vi "SelectPage2.vi"(8 "error in (no error)":errorcluster, 11 "Controller in":refnum<class "Controller.lvclass">) -> (0 "error out":errorcluster, 3 "Controller out":refnum<class "Controller.lvclass">)   [LabVIEW 2020, in "Container.lvlib" / "Controller.lvclass"]
uses:
  Controller.lvclass
  Controller.lvclass/Controller.ctl
  Page2/View/View.lvclass
  C:/Users/N Tan/Documents/2-Prototypes/MVC-Multi-Page/iView/iView.lvclass
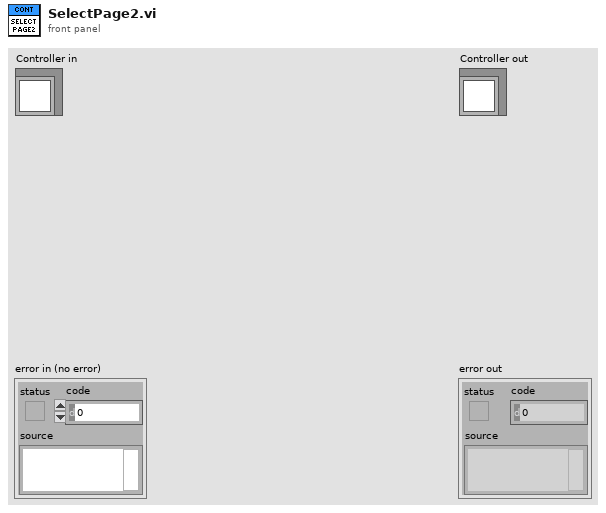
[diagram p1: front panel]
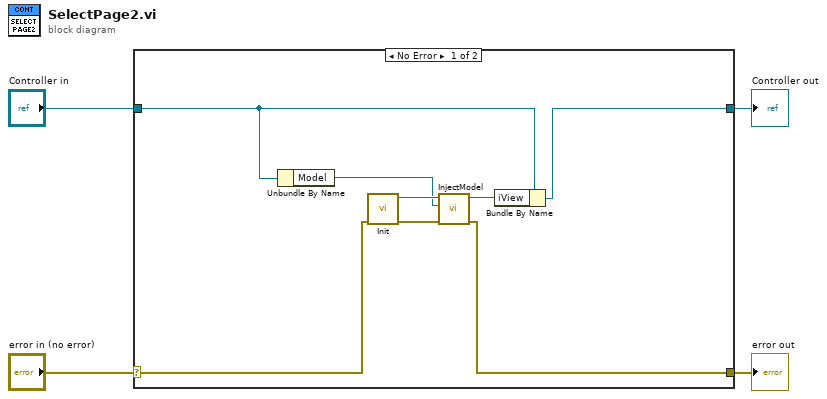
[diagram p0: block diagram]
diagram:
  n1 = case shown="No Error" "error in (no error)" {
    selector: "error in (no error)" -> [w11 w14]
    tunnel: [w7 w14] -> w3
    tunnel: [w12 w13] -> w1
    tunnel: "Controller in" -> [w6 w13]
    frame No Error {
      n2 = Unbundle By Name(w6) -> ("Model"=w5:refnum<class "Model.lvclass">)
      n3 = call "Init.vi"("error in (no error)"=w11) -> ("error out"=w8:errorcluster, "View out"=w10:refnum<class "View.lvclass">)  [unwired: 9 in]
      n4 = call "InjectModel.vi"("error in (no error)"=w8, "Model"=w5, "View in"=w10) -> ("error out"=w7:errorcluster, "View out"=w9:refnum<class "View.lvclass">)  [unwired: 7 in]
      n5 = Bundle By Name(cluster=w6, "iView"=w9) -> (w12:refnum<class "Controller.lvclass">)
    }
    frame Error {
    }
  }
  "error out" <- w3
  "Controller out" <- w1
